vi "Read_Raw.vi"(8 "error in (no error)":errorcluster, 11 "BMP208 in":refnum<class "BMP208.lvclass">) -> (0 "error out":errorcluster, 1 "PressureU32":u32 format="%020b", 2 "TempU32":u32 format="%020b", 3 "BMP208 out":refnum<class "BMP208.lvclass">)   [LabVIEW 2020, in "BMP208.lvclass"]
uses:
  BMP208.lvclass
  LINX I2C/LINX I2C.lvclass
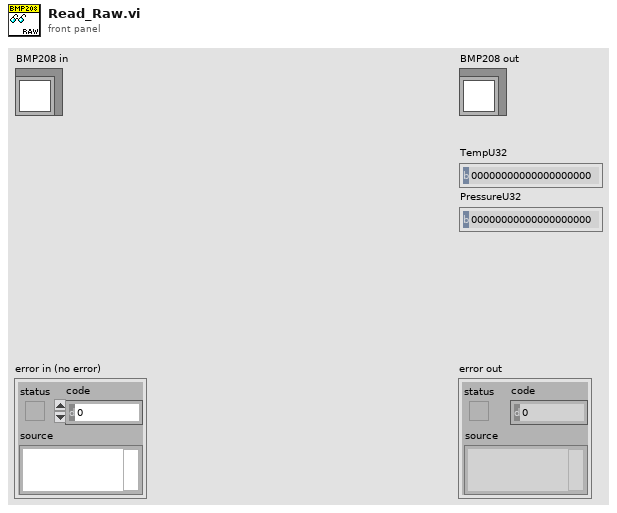
[diagram p1: front panel]
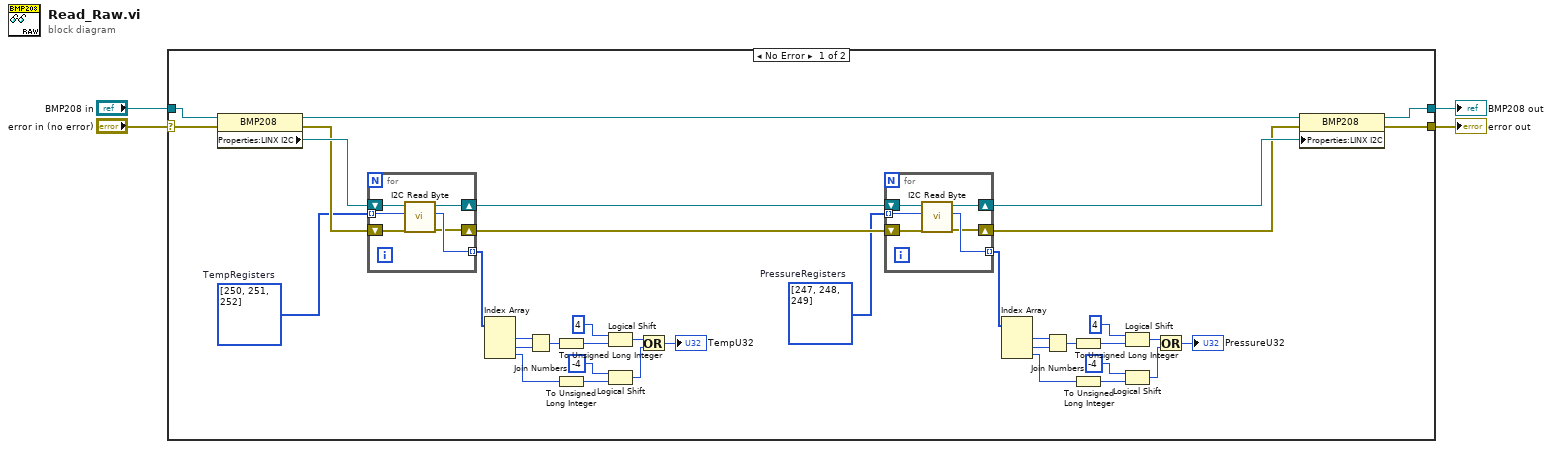
[diagram p0: block diagram]
diagram:
  n1 = case shown="No Error" "error in (no error)" {
    selector: "error in (no error)" -> [w41 w55]
    tunnel: [w37 w55] -> w3
    tunnel: [w38 w54] -> w1
    tunnel: "BMP208 in" -> [w40 w54]
    frame No Error {
      w7 = u8[] [247, 248, 249]  # PressureRegisters
      w22 = u8[] [250, 251, 252]  # TempRegisters
      n2 = property class="BMP208"(reference=w40, error in=w41) -> (reference out=w39:refnum<class "BMP208.lvclass">, error out=w23:errorcluster, "Properties:LINX I2C"=w24:refnum<class "LINX I2C.lvclass">)
      n3 = for {
        tunnel: w22 -> [w51] mode=indexing
        tunnel: [w50] -> w30 mode=indexing
        shift-right: [w49] -> w9
        shift-left: w24 -> [w53]
        shift-right: [w48] -> w8
        shift-left: w23 -> [w52]
        n4 = call-dynamic "I2C Read Byte.vi"("error in (no error)"=w52, "Register Address"=w51, "LINX I2C in"=w53) -> ("error out"=w48:errorcluster, "Byte Read"=w50:u8, "LINX I2C out"=w49:refnum<class "LINX I2C.lvclass">)  [unwired: 6 in]
      }
      n5 = Index Array(array=w30) -> (element #1=w29:u8, element #2=w28:u8, element #3=w27:u8)  [unwired: 3 in]
      n6 = Join Numbers(hi=w29, lo=w28) -> ((hi.lo)=w31:u16)
      n7 = To Unsigned Long Integer(number=w31) -> (unsigned 32bit integer=w33:u32)
      n8 = To Unsigned Long Integer(number=w27) -> (unsigned 32bit integer=w34:u32)
      n9 = Logical Shift(y=i16 4, x=w33) -> (x << y=w32:u32)
      n10 = Logical Shift(y=i16 -4, x=w34) -> (x << y=w35:u32)
      n11 = Or(x=w32, y=w35) -> (x .or. y?=→"TempU32":u32)
      n12 = for {
        tunnel: w7 -> [w45] mode=indexing
        tunnel: [w44] -> w16 mode=indexing
        shift-right: [w43] -> w6
        shift-left: w9 -> [w47]
        shift-right: [w42] -> w5
        shift-left: w8 -> [w46]
        n13 = call-dynamic "I2C Read Byte.vi"("error in (no error)"=w46, "Register Address"=w45, "LINX I2C in"=w47) -> ("error out"=w42:errorcluster, "Byte Read"=w44:u8, "LINX I2C out"=w43:refnum<class "LINX I2C.lvclass">)  [unwired: 6 in]
      }
      n14 = Index Array(array=w16) -> (element #1=w17:u8, element #2=w18:u8, element #3=w19:u8)  [unwired: 3 in]
      n15 = Join Numbers(hi=w17, lo=w18) -> ((hi.lo)=w15:u16)
      n16 = To Unsigned Long Integer(number=w15) -> (unsigned 32bit integer=w13:u32)
      n17 = To Unsigned Long Integer(number=w19) -> (unsigned 32bit integer=w12:u32)
      n18 = Logical Shift(y=i16 4, x=w13) -> (x << y=w14:u32)
      n19 = Logical Shift(y=i16 -4, x=w12) -> (x << y=w11:u32)
      n20 = Or(x=w14, y=w11) -> (x .or. y?=→"PressureU32":u32)
      n21 = property class="BMP208"(reference=w39, error in=w5, "Properties:LINX I2C"=w6) -> (reference out=w38:refnum<class "BMP208.lvclass">, error out=w37:errorcluster)
    }
    frame Error {
    }
  }
  "error out" <- w3
  "BMP208 out" <- w1
